vi "Open VI Reference.vi"(8 "Error In":errorcluster, 11 "VI Info":T1) -> (0 "Error Out":errorcluster, 3 "VI":refnum<vi>)   [LabVIEW 2017, in "Bookmark Manager.lvlib"]
uses:
  Bookmark Manager.lvlib
  Controls/VI Information.ctl
  Controls/Application Information.ctl
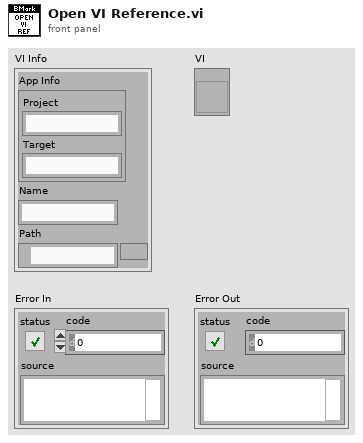
[diagram p1: front panel]
types:
  T1 = typedef "Bookmark Manager.lvlib/VI Information.ctl" = cluster{"App Info":T2, "Name":string, "Path":path}
  T2 = typedef "Bookmark Manager.lvlib/Application Information.ctl" = cluster{"Project":string, "Target":string}
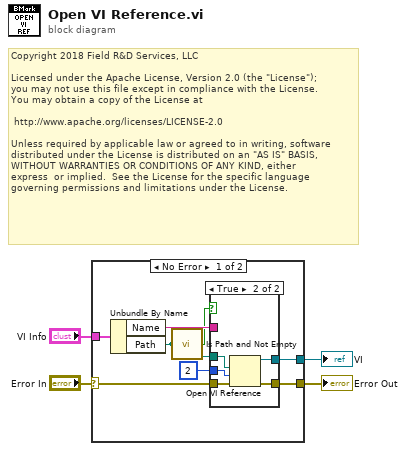
[diagram p0: block diagram]
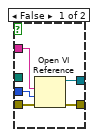
[diagram p2: hidden frame]
diagram:
  # "Copyright 2018 Field R&D Services, LLC\n\nLicensed under the Apache License, Version 2.0 (the \"License\");\nyou may not use this file except in compliance with the License.\nYou may obtain a copy of the License at\n\n\thttp://www.apache.org/licenses/LICENSE-2.0\n\nUnless required by applicable law or agreed to in writing, software\ndistributed under the License is distributed on an \"AS IS\" BASIS,\nWITHOUT WARRANTIES OR CONDITIONS OF ANY KIND, either \nexpress  or implied.  See the License for the specific language \ngoverning permissions and limitations under the License."
  n1 = case shown="No Error" "Error In" {
    selector: "Error In" -> [w5 w23]
    tunnel: "VI Info" -> [w9 _]
    tunnel: [w8 _] -> w3
    tunnel: [w7 w23] -> w2
    frame No Error {
      n2 = Unbundle By Name(w9) -> ("Name"=w12:string, "Path"=w11:path)
      n3 = call <vilib>:"Is Path and Not Empty.vi"("path"=w11) -> ("Is Path and Not Empty?"=w10:bool)  [unwired: 4 in]
      n4 = case shown="True" w10 {
        tunnel: [w16 w22] -> w7
        tunnel: [w14 w21] -> w8
        tunnel: w5 -> [w17 w20]
        tunnel: w11 -> [_ w19]
        tunnel: w12 -> [w15 _]
        tunnel: 2 ("options") -> [w13 w18]
        frame False {
          n5 = Open VI Reference(vi path=w15, options=w13, error in (no error)=w17) -> (vi reference=w14:refnum<vi>, error out=w16:errorcluster)  [unwired: 3 in]
        }
        frame True {
          n6 = Open VI Reference(vi path=w19, options=w18, error in (no error)=w20) -> (vi reference=w21:refnum<vi>, error out=w22:errorcluster)  [unwired: 3 in]
        }
      }
    }
    frame Error {
    }
  }
  "VI" <- w3
  "Error Out" <- w2
